vi "serpenbot_DDPG_control_parallel_old_camera_2.vi"() -> ()   [LabVIEW 2020]
uses:
  <vilib>/Analysis/Matrix/Datatypes/RealMatrix.ctl
  <vilib>/Analysis/Matrix/NI_Matrix.lvlib
  <vilib>/Analysis/NI_AALPro.lvlib
  <vilib>/Analysis/_algsub.llb/Real PseudoInverse Matrix.vi
  <vilib>/Analysis/NI_AALBase.lvlib
  <vilib>/Analysis/baseanly.llb/Real A x B.vi
  <vilib>/Analysis/Matrix/Numeric/Subtract/Subtract - RM,RM.vi
panel:
  out "camera_value 2":T1
  out "appended array 3":T1
  out "error out Y":errorcluster
  out "error out X":errorcluster
  in  "goal y":dbl
  in  "goal x":dbl
  in  "k":T1
  out "control_loop_time":u32
  in  "stop":bool
  in  "Logging":bool caption="Enable"
  out "current x":dbl
  out "current y":dbl
  out "laser control value":dbl[](array[numeric])
  in  "Diode Current\nSetting":dbl=3.0
  in  "Laser Repetition\nFrequency":i32=50000
  in  "VISA resource name":refnum<visa-resource-name>="COM14"
  in  "baud rate (9600)":u32=9600
  out "error out":errorcluster
  out "Identification system 1":string
  out "Conn. axes system 1":string[](array[string])
  out "Identification system 2":string
  out "Conn. axes system  2":string[](array[string])
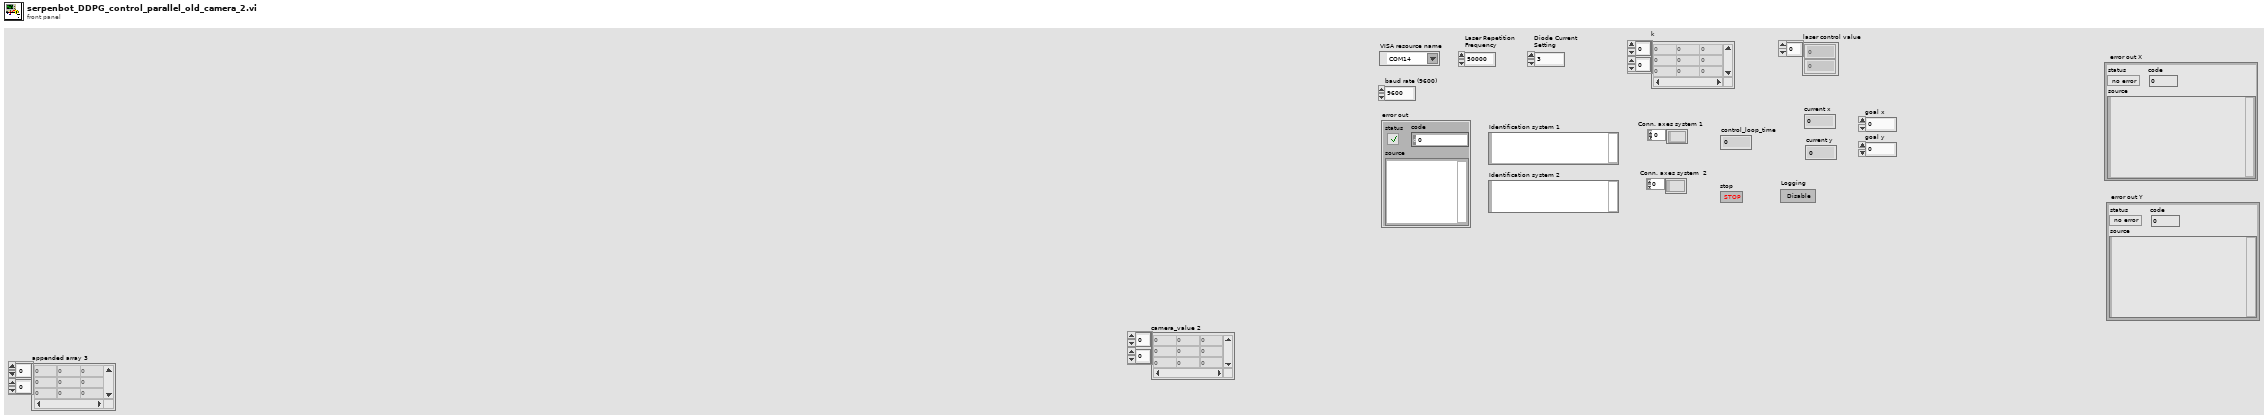
[diagram p1: front panel]
types:
  T1 = typedef "NI_Matrix.lvlib/RealMatrix.ctl" = dbl[][]
  T2 = cluster{"RS232 settings":cluster{"Portnumber":i32, "Baudrate":u16}, "USB settings":cluster{"S/N":string, "USB Search?":bool}, "TCP/IP settings":cluster{"Host address/name":string, "Port":i32, "Board":i32, "TCP/IP Search?":bool}}
  T3 = cluster{"Check FRF?":bool, "Referencing mode":enum16{"FRF (-> FNL)", "FRF", "FNL", "FPL", "RON OFF"}[]}
  T4 = cluster{"Force?":bool, "Dialog?":bool, "Stages":string[]}
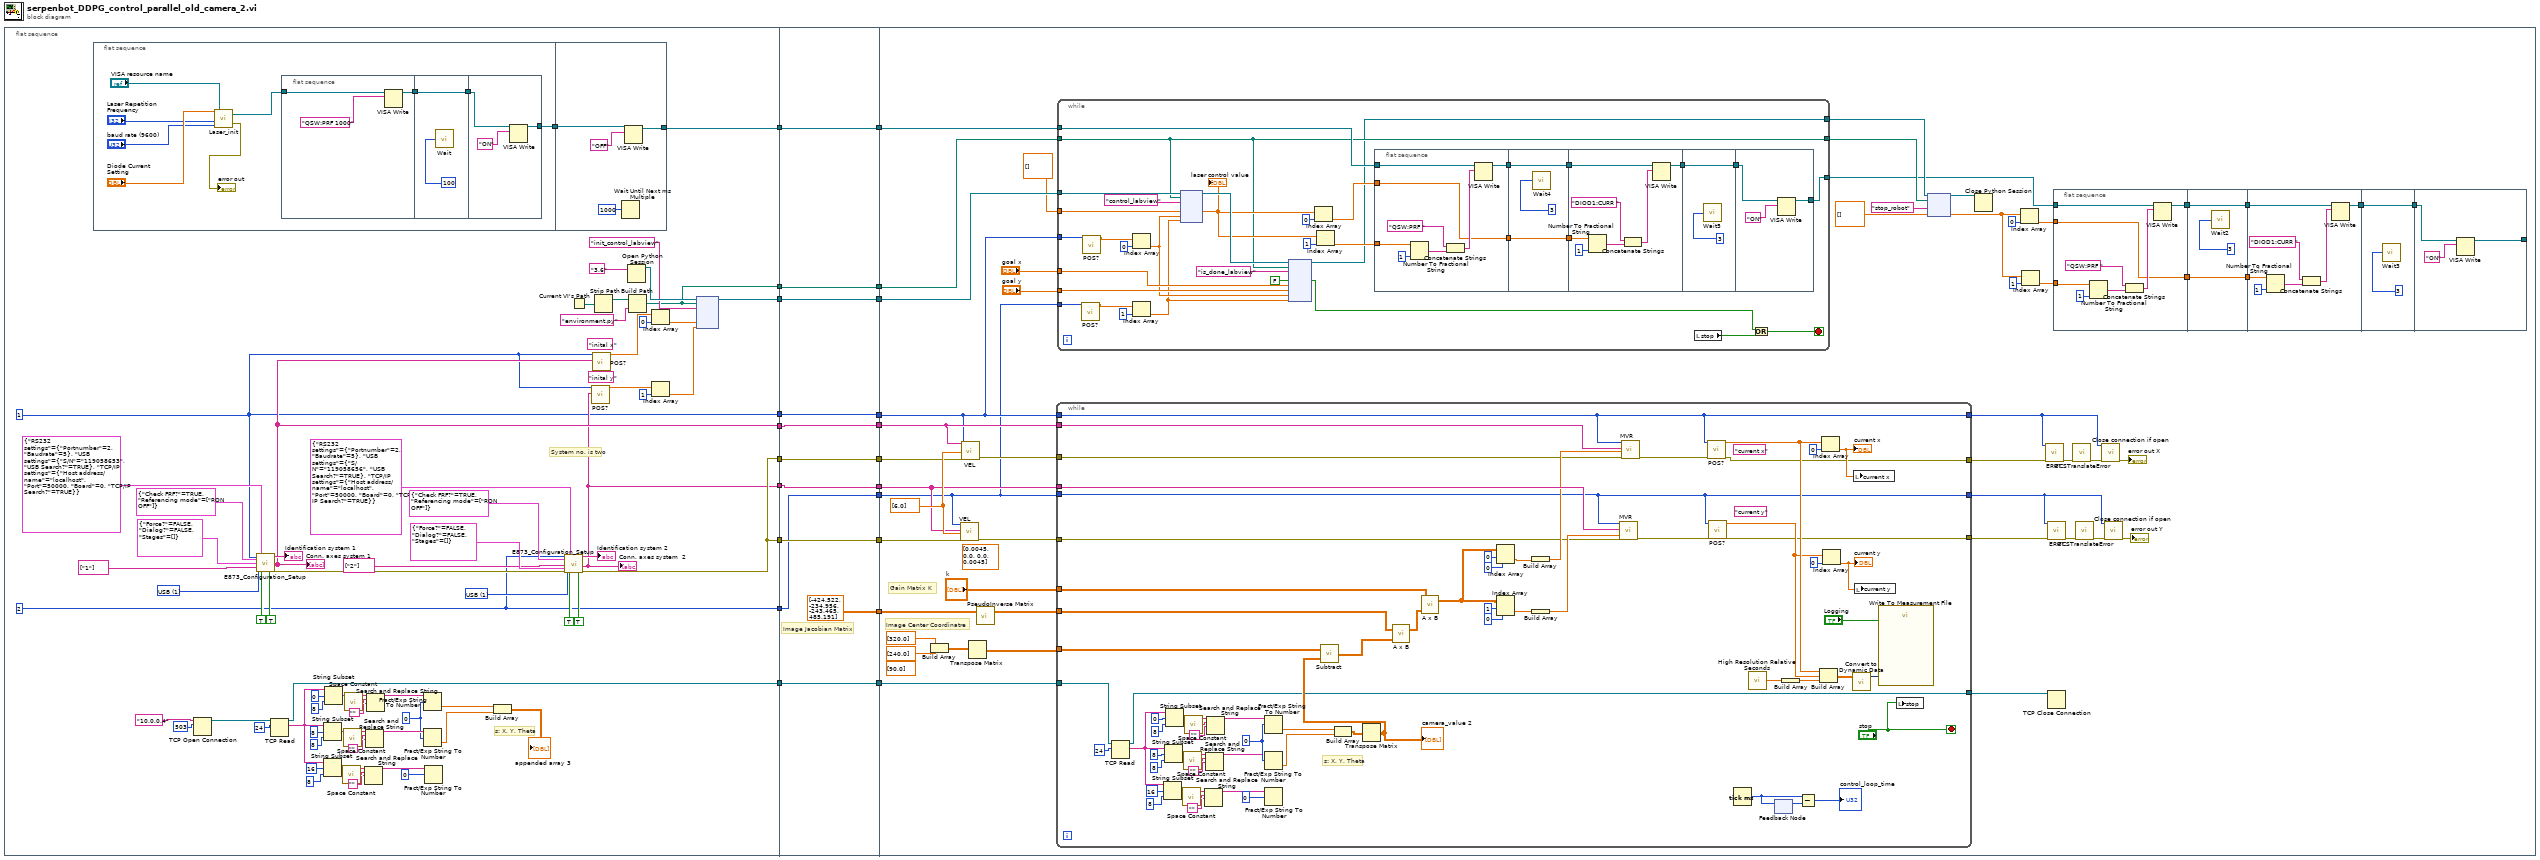
[diagram p0: block diagram]
diagram:
  n1 = flat-sequence {
    tunnel: [w87] -> w21
    tunnel: [w57] -> w20
    tunnel: [w59] -> w19
    tunnel: [w68] -> w18
    tunnel: [w58] -> w17
    tunnel: [w69] -> w16
    tunnel: [w68] -> w15
    tunnel: [w61] -> w14
    tunnel: [w60] -> w13
    tunnel: [w22] -> w1
    tunnel: w21 -> [w120]
    tunnel: [w120] -> w12
    tunnel: w20 -> [w119]
    tunnel: w19 -> [w118]
    tunnel: w18 -> [w117]
    tunnel: w17 -> [w116]
    tunnel: w16 -> [w114]
    tunnel: [w119] -> w11
    tunnel: [w118] -> w10
    tunnel: [w117] -> w9
    tunnel: [w116] -> w8
    tunnel: w15 -> [w115]
    tunnel: [w115] -> w7
    tunnel: [w114] -> w6
    tunnel: [T1 [[-424.522, -234.956], [-243.465, 485.191]] ("J_init 2")] -> w5
    tunnel: w14 -> [w112]
    tunnel: w13 -> [w111]
    tunnel: [w112] -> w4
    tunnel: [w111] -> w3
    tunnel: [w110] -> w2
    tunnel: w1 -> [w110]
    tunnel: w12 -> [w141]
    tunnel: w11 -> [w122]
    tunnel: w10 -> [w164]
    tunnel: w9 -> [w167]
    tunnel: w8 -> [w162]
    tunnel: w7 -> [w166]
    tunnel: w6 -> [w121]
    tunnel: w5 -> [w165]
    tunnel: w4 -> [w143]
    tunnel: w3 -> [w142]
    tunnel: w2 -> [w124]
    frame #0 {
      w36 = 0
      (unwired) "inital y"
      (unwired) "inital x"
      w72 = u16 1 items=["RS232", "USB", "TCP/IP"] ("Interface")
      w75 = u16 1 items=["RS232", "USB", "TCP/IP"] ("Interface")
      w69 = 2 ("System no.")
      w57 = 1 ("System no.")
      # "s: X, Y, Theta"
      # "System no. is two"
      n2 = flat-sequence {
        tunnel: [w89] -> w88
        tunnel: w88 -> [w107]
        tunnel: [w106] -> w87
        frame #0 {
          n3 = call "Laser_init.vi"("baud rate (9600)"="baud rate (9600)", "Laser Repetition\nFrequency"="Laser Repetition\nFrequency", "VISA resource name"="VISA resource name", "Diode Current\nSetting"="Diode Current\nSetting") -> ("error out"=→"error out":errorcluster, "VISA Refnum out"=w90:refnum<visa-resource-name>)
          n4 = flat-sequence {
            tunnel: w90 -> [w100]
            tunnel: [w99] -> w97
            tunnel: w97 -> [w102]
            tunnel: [w102] -> w96
            tunnel: w96 -> [w103]
            tunnel: [w104] -> w89
            frame #0 {
              n5 = VISA Write(VISA resource name=w100, write buffer="QSW:PRF 1000" ("string")) -> (VISA resource name out=w99:refnum<visa-resource-name>)  [unwired: 1 in, 2 out]
            }
            frame #1 {
              n6 = call "Wait"("Count(mSec)"=u32 100) -> ()  [unwired: 1 out]
            }
            frame #2 {
              n7 = VISA Write(VISA resource name=w103, write buffer="ON") -> (VISA resource name out=w104:refnum<visa-resource-name>)  [unwired: 1 in, 2 out]
            }
          }
        }
        frame #1 {
          n8 = Wait Until Next ms Multiple(millisecond multiple=u32 1000) -> ()  [unwired: 1 out]
          n9 = VISA Write(VISA resource name=w107, write buffer="OFF") -> (VISA resource name out=w106:refnum<visa-resource-name>)  [unwired: 1 in, 2 out]
        }
      }
      n10 = TCP Open Connection(address="10.0.0.4", remote port or service name=u16 503) -> (connection ID=w46:refnum<k5>)  [unwired: 3 in, 1 out]
      n11 = call "E873_Configuration_Setup.vi"("System no."=w57, "Referencing"=T3 {"Check FRF?"=TRUE, "Referencing mode"=[enum."RON OFF"]}, "Interface"=w75, "All axes?"=TRUE, "Axes to move"=string[] ["1"], "Interface settings"=T2 {"RS232 settings"={"Portnumber"=2, "Baudrate"=5}, "USB settings"={"S/N"="119058653", "USB Search?"=TRUE}, "TCP/IP settings"={"Host address/name"="localhost", "Port"=50000, "Board"=0, "TCP/IP Search?"=TRUE}}, "Stage selection"=T4 {"Force?"=FALSE, "Dialog?"=FALSE, "Stages"=[]}, "Switch servo on?"=TRUE ("Use dialog to define\nconnected stages?")) -> ("Identification"=→"Identification system 1":string, "Conn. \nAxes"=w59:string[], "error out"=w84:errorcluster)  [unwired: 4 in, 5 out]
      "Conn. axes system 1" <- w59
      n12 = TCP Read(connection ID=w46, bytes to read=24) -> (connection ID out=w22:refnum<k5>, data out=w45:string)  [unwired: 3 in, 1 out]
      n13 = String Subset(string=w45, offset (0)=16, length (rest)=8 ("length (rest)")) -> (substring=w43:string)
      n14 = String Subset(string=w45, offset (0)=8, length (rest)=8 ("length (rest)")) -> (substring=w44:string)
      n15 = String Subset(string=w45, offset (0)=0, length (rest)=8 ("length (rest)")) -> (substring=w42:string)
      n16 = call <vilib>:"Space Constant.vi"() -> ("String"=w41:string)
      n17 = call <vilib>:"Space Constant.vi"() -> ("String"=w40:string)
      n18 = call <vilib>:"Space Constant.vi"() -> ("String"=w39:string)
      n19 = Search and Replace String(input string=w43, search string=w41, replace string="") -> (result string=w47:string)  [unwired: 5 in, 3 out]
      n20 = Search and Replace String(input string=w44, search string=w40, replace string="") -> (result string=w48:string)  [unwired: 5 in, 3 out]
      n21 = Search and Replace String(input string=w42, search string=w39, replace string="") -> (result string=w49:string)  [unwired: 5 in, 3 out]
      n22 = Fract/Exp String To Number(string=w49, offset=w36) -> (number=w37:dbl)  [unwired: 2 in, 1 out]
      n23 = Fract/Exp String To Number(string=w48, offset=w36) -> (number=w38:dbl)  [unwired: 2 in, 1 out]
      n24 = Fract/Exp String To Number(string=w47, offset=0) -> ()  [unwired: 2 in, 2 out]
      n25 = Build Array(w37, w38) -> (→"appended array 3":T1)
      n26 = call "E873_Configuration_Setup.vi"("System no."=w69, "Referencing"=T3 {"Check FRF?"=TRUE, "Referencing mode"=[enum."RON OFF"]}, "Interface"=w72, "All axes?"=TRUE, "Axes to move"=string[] ["2"], "error in"=w84, "Interface settings"=T2 {"RS232 settings"={"Portnumber"=2, "Baudrate"=5}, "USB settings"={"S/N"="119058656", "USB Search?"=TRUE}, "TCP/IP settings"={"Host address/name"="localhost", "Port"=50000, "Board"=0, "TCP/IP Search?"=TRUE}}, "Stage selection"=T4 {"Force?"=FALSE, "Dialog?"=FALSE, "Stages"=[]}, "Switch servo on?"=TRUE ("Use dialog to define\nconnected stages?")) -> ("Identification"=→"Identification system 2":string, "Conn. \nAxes"=w58:string[], "error out"=w68:errorcluster)  [unwired: 3 in, 5 out]
      "Conn. axes system  2" <- w58
      n27 = Current VI's Path() -> (path=w67:path)
      n28 = call "POS?.vi"("System no."=w57, "Axes to query"=w58) -> ("Position"=w52:dbl[])  [unwired: 3 in, 14 out]
      n29 = call "POS?.vi"("System no."=w57, "Axes to query"=w59) -> ("Position"=w54:dbl[])  [unwired: 3 in, 14 out]
      n30 = Strip Path(path=w67) -> (stripped path=w66:path)  [unwired: 1 out]
      n31 = Open Python Session(python version="3.6" ("Python version")) -> (session out=w63:refnum<k35>)  [unwired: 2 in, 1 out]
      n32 = Build Path(base path=w66, name or relative path="environment.py") -> (appended path=w61:path)
      n33 = Index Array(array=w54, index=0) -> (element=w55:dbl)
      n34 = Index Array(array=w52, index=1) -> (element=w51:dbl)
      n35 = node(w63, w61, "init_control_labview" ("function name"), w55, w51) -> (w60:refnum<k35>)  [unwired: 5 in, 3 out]
    }
    frame #1 {
      # "Image Jacobian Matrix"
    }
    frame #2 {
      w168 = dbl[] [6.0] ("Velocity values")
      (unwired) T1 [[0.0045, 0.0], [0.0, 0.0045]] ("J_init 2")
      (unwired) dbl[] [90.0] ("element")
      # "Gain Matrix K"
      # "Image Center Coordinatre"
      n36 = Build Array(dbl[] [320.0] ("element"), dbl[] [240.0] ("element")) -> (w169:T1)
      n37 = call "VEL.vi"("System no."=w121, "Axes to set"=w162, "Velocity values"=w168, "error in"=w166) -> ("error out"=w161:errorcluster)  [unwired: 2 in, 13 out]
      n38 = call "VEL.vi"("System no."=w122, "Axes to set"=w164, "Velocity values"=w168, "error in"=w167) -> ("error out"=w163:errorcluster)  [unwired: 2 in, 13 out]
      n39 = Transpose Matrix(1:w169) -> (0:w158:T1)
      n40 = call-poly <vilib>:"PseudoInverse Matrix.vi"("Input Matrix"=w165) -> ("PseudoInverse Matrix"=w159:T1)  [unwired: 1 in, 1 out]
      n41 = while {
        tunnel: w161 -> [w277]
        tunnel: w121 -> [w258]
        tunnel: w162 -> [w295]
        tunnel: w163 -> [w278]
        tunnel: w164 -> [w294]
        tunnel: w122 -> [w260]
        tunnel: w159 -> [w283]
        tunnel: "k" -> [w282]
        tunnel: w158 -> [w281]
        tunnel: [w260] -> w127
        tunnel: [w259] -> w128
        tunnel: [w258] -> w126
        tunnel: [w257] -> w125
        tunnel: w124 -> [w230]
        tunnel: [w229] -> w123
        stop <- "stop" stop-if-true
        w256 = 0
        (unwired) "current y"
        (unwired) "current x"
        # "s: X, Y, Theta"
        n42 = TCP Read(connection ID=w230, bytes to read=24) -> (connection ID out=w229:refnum<k5>, data out=w237:string)  [unwired: 3 in, 1 out]
        n43 = String Subset(string=w237, offset (0)=16, length (rest)=8 ("length (rest)")) -> (substring=w239:string)
        n44 = String Subset(string=w237, offset (0)=8, length (rest)=8 ("length (rest)")) -> (substring=w238:string)
        n45 = String Subset(string=w237, offset (0)=0, length (rest)=8 ("length (rest)")) -> (substring=w244:string)
        n46 = call <vilib>:"Space Constant.vi"() -> ("String"=w247:string)
        n47 = call <vilib>:"Space Constant.vi"() -> ("String"=w249:string)
        n48 = call <vilib>:"Space Constant.vi"() -> ("String"=w251:string)
        n49 = Search and Replace String(input string=w239, search string=w247, replace string="") -> (result string=w235:string)  [unwired: 5 in, 3 out]
        n50 = Search and Replace String(input string=w238, search string=w249, replace string="") -> (result string=w234:string)  [unwired: 5 in, 3 out]
        n51 = Search and Replace String(input string=w244, search string=w251, replace string="") -> (result string=w233:string)  [unwired: 5 in, 3 out]
        n52 = Fract/Exp String To Number(string=w233, offset=w256) -> (number=w255:dbl)  [unwired: 2 in, 1 out]
        n53 = Fract/Exp String To Number(string=w234, offset=w256) -> (number=w254:dbl)  [unwired: 2 in, 1 out]
        n54 = Fract/Exp String To Number(string=w235, offset=0) -> ()  [unwired: 2 in, 2 out]
        n55 = Build Array(w255, w254) -> (w232:T1)
        n56 = Transpose Matrix(1:w232) -> (0:w231:T1)
        "camera_value 2" <- w231
        n57 = call-poly <vilib>:"Subtract.vi"("Real Matrix B"=w231, "Real Matrix A"=w281) -> ("A - B"=w289:T1)
        n58 = call-poly <vilib>:"A x B.vi"("B"=w289, "A"=w283) -> ("A x B"=w287:T1)  [unwired: 1 out]
        n59 = call-poly <vilib>:"A x B.vi"("B"=w287, "A"=w282) -> ("A x B"=w288:T1)  [unwired: 1 out]
        n60 = Index Array(array=w288, index (row)=0, index (col)=0) -> (element=w280:dbl)
        n61 = Index Array(array=w288, index (row)=1, index (col)=0) -> (element=w279:dbl)
        n62 = Build Array(w280) -> (w286:dbl[])
        n63 = Build Array(w279) -> (w285:dbl[])
        n64 = call "MVR.vi"("System no."=w258, "Axes to move"=w295, "Position values"=w285, "error in"=w277) -> ("error out"=w269:errorcluster)  [unwired: 1 in, 14 out]
        n65 = call "MVR.vi"("System no."=w260, "Axes to move"=w294, "Position values"=w286, "error in"=w278) -> ("error out"=w270:errorcluster)  [unwired: 1 in, 14 out]
        n66 = call "POS?.vi"("System no."=w260, "error in"=w270) -> ("Position"=w267:dbl[], "error out"=w259:errorcluster)  [unwired: 3 in, 13 out]
        n67 = call "POS?.vi"("System no."=w258, "error in"=w269) -> ("Position"=w265:dbl[], "error out"=w257:errorcluster)  [unwired: 3 in, 13 out]
        n68 = Tick Count (ms)() -> (millisecond timer value=w268:u32)
        n69 = call <vilib>:"High Resolution Relative Seconds.vi"() -> ("relative seconds"=w272:dbl)
        n70 = feedback #1() -> (w284:u32)  [unwired: 1 in]
        n71 = feedback-in #1(w268) -> ()
        n72 = Build Array(w272) -> (w271:dbl[])
        n73 = Subtract(x=w268, y=w284) -> (x-y=→"control_loop_time":u32)
        n74 = Build Array(w267, w265, w271) -> (w274:dbl[][])
        n75 = Index Array(array=w267, index=0) -> (element=w263:dbl)
        "current x" <- w263
        n76 = Index Array(array=w265, index=0) -> (element=w262:dbl)
        "current y" <- w262
        n77 = call "Convert to Dynamic Data"("2D Array"=w274) -> ("Dynamic Data Type"=w273:dynamicdata)  [unwired: 3 in]
        n78 = local write "current x"(w263) -> ()
        n79 = local write "current y"(w262) -> ()
        n80 = call "Write To Measurement File"("Signals"=w273, "Enable"="Logging") -> ()  [unwired: 15 in, 3 out]
        n81 = local write "stop"("stop") -> ()
      }
      n82 = while {
        tunnel: dbl[] [] -> [w190]
        tunnel: "goal x" -> [w189]
        tunnel: "goal y" -> [w188]
        tunnel: w143 -> [w185]
        tunnel: w142 -> [w187]
        tunnel: w141 -> [w186]
        tunnel: [w185] -> w140
        tunnel: [w184] -> w139
        tunnel: [w181] -> w138
        tunnel: w122 -> [w179]
        tunnel: w121 -> [w172]
        stop <- w182 stop-if-true
        n83 = call "POS?.vi"("System no."=w172) -> ("Position"=w174:dbl[])  [unwired: 4 in, 14 out]
        n84 = call "POS?.vi"("System no."=w179) -> ("Position"=w177:dbl[])  [unwired: 4 in, 14 out]
        n85 = Index Array(array=w174, index=1) -> (element=w173:dbl)
        n86 = Index Array(array=w177, index=0) -> (element=w176:dbl)
        n87 = node(w187, w185, "control_labview" ("function name"), w190, w176, w173) -> (w198:refnum<k35>, w192:dbl[])  [unwired: 3 in, 3 out]
        "laser control value" <- w192
        n88 = node(w198, w185, "is_done_labview" ("function name"), FALSE, w189, w188, w176, w173) -> (w184:refnum<k35>, w180:bool)  [unwired: 5 in, 3 out]
        n89 = Index Array(array=w192, index=0) -> (element=w195:dbl)
        n90 = Index Array(array=w192, index=1) -> (element=w191:dbl)
        n91 = flat-sequence {
          tunnel: w186 -> [w209]
          tunnel: [w208] -> w205
          tunnel: w191 -> [w207]
          tunnel: w195 -> [w206]
          tunnel: [w206] -> w204
          tunnel: [w216] -> w203
          tunnel: [w214] -> w202
          tunnel: w205 -> [w216]
          tunnel: w204 -> [w214]
          tunnel: [w223] -> w201
          tunnel: w203 -> [w221]
          tunnel: w202 -> [w218]
          tunnel: w201 -> [w225]
          tunnel: [w225] -> w200
          tunnel: w200 -> [w227]
          tunnel: [w226] -> w181
          frame #0 {
            n92 = Number To Fractional String(number=w207, precision (6)=i16 1) -> (F-format string=w212:string)  [unwired: 2 in]
            n93 = Concatenate Strings("QSW:PRF " ("string"), w212) -> (w213:string)
            n94 = VISA Write(VISA resource name=w209, write buffer=w213) -> (VISA resource name out=w208:refnum<visa-resource-name>)  [unwired: 1 in, 2 out]
          }
          frame #1 {
            n95 = call "Wait4"("Count(mSec)"=u32 3) -> ()  [unwired: 1 out]
          }
          frame #2 {
            n96 = Number To Fractional String(number=w218, precision (6)=i16 1) -> (F-format string=w219:string)  [unwired: 2 in]
            n97 = Concatenate Strings("DIOD1:CURR " ("string"), w219) -> (w222:string)
            n98 = VISA Write(VISA resource name=w221, write buffer=w222) -> (VISA resource name out=w223:refnum<visa-resource-name>)  [unwired: 1 in, 2 out]
          }
          frame #3 {
            n99 = call "Wait5"("Count(mSec)"=u32 3) -> ()  [unwired: 1 out]
          }
          frame #4 {
            n100 = VISA Write(VISA resource name=w227, write buffer="ON") -> (VISA resource name out=w226:refnum<visa-resource-name>)  [unwired: 1 in, 2 out]
          }
        }
        n101 = local read "stop"() -> (w183:bool)
        n102 = Or(x=w180, y=w183) -> (x .or. y?=w182:bool)
      }
      n103 = node(w139, w140, "stop_robot" ("function name"), dbl[] []) -> (w149:refnum<k35>, w144:dbl[])  [unwired: 1 in, 3 out]
      n104 = Close Python Session(session in=w149) -> ()  [unwired: 1 in, 1 out]
      n105 = Index Array(array=w144, index=0) -> (element=w146:dbl)
      n106 = Index Array(array=w144, index=1) -> (element=w145:dbl)
      n107 = call "ERR?.vi"("System no."=w127, "error in"=w128) -> ("error out"=w132:errorcluster)  [unwired: 17 out]
      n108 = call "ERR?.vi"("System no."=w126, "error in"=w125) -> ("error out"=w129:errorcluster)  [unwired: 17 out]
      n109 = TCP Close Connection(connection ID=w123) -> ()  [unwired: 2 in, 2 out]
      n110 = flat-sequence {
        tunnel: w138 -> [w299]
        tunnel: [w298] -> w157
        tunnel: w145 -> [w297]
        tunnel: w146 -> [w296]
        tunnel: [w296] -> w156
        tunnel: [w306] -> w155
        tunnel: [w304] -> w154
        tunnel: w157 -> [w306]
        tunnel: w156 -> [w304]
        tunnel: [w313] -> w153
        tunnel: w155 -> [w311]
        tunnel: w154 -> [w308]
        tunnel: w153 -> [w315]
        tunnel: [w315] -> w152
        tunnel: w152 -> [w317]
        tunnel: [w316] -> _
        frame #0 {
          n111 = Number To Fractional String(number=w297, precision (6)=i16 1) -> (F-format string=w302:string)  [unwired: 2 in]
          n112 = Concatenate Strings("QSW:PRF " ("string"), w302) -> (w303:string)
          n113 = VISA Write(VISA resource name=w299, write buffer=w303) -> (VISA resource name out=w298:refnum<visa-resource-name>)  [unwired: 1 in, 2 out]
        }
        frame #1 {
          n114 = call "Wait2"("Count(mSec)"=u32 3) -> ()  [unwired: 1 out]
        }
        frame #2 {
          n115 = Number To Fractional String(number=w308, precision (6)=i16 1) -> (F-format string=w309:string)  [unwired: 2 in]
          n116 = Concatenate Strings("DIOD1:CURR " ("string"), w309) -> (w312:string)
          n117 = VISA Write(VISA resource name=w311, write buffer=w312) -> (VISA resource name out=w313:refnum<visa-resource-name>)  [unwired: 1 in, 2 out]
        }
        frame #3 {
          n118 = call "Wait3"("Count(mSec)"=u32 3) -> ()  [unwired: 1 out]
        }
        frame #4 {
          n119 = VISA Write(VISA resource name=w317, write buffer="ON") -> (VISA resource name out=w316:refnum<visa-resource-name>)  [unwired: 1 in, 2 out]
        }
      }
      n120 = call "GCSTranslateError.vi"("error in"=w132) -> ("error out"=w133:errorcluster)  [unwired: 18 out]
      n121 = call "GCSTranslateError.vi"("error in"=w129) -> ("error out"=w130:errorcluster)  [unwired: 18 out]
      n122 = call "Close connection if open.vi"("System no."=w127, "error in"=w133) -> ("error out"=→"error out X":errorcluster)  [unwired: 1 in, 16 out]
      n123 = call "Close connection if open.vi"("System no."=w126, "error in"=w130) -> ("error out"=→"error out Y":errorcluster)  [unwired: 1 in, 16 out]
    }
  }
